vi "TangoEventsTest.vi"() -> ()   [LabVIEW 2009]
uses:
  tango_lv9/tango_vi.llb/tango.lvlib
  tango_lv9/tango_vi.llb/toShortScalar.vi
panel:
  in  "event timeout (ms)":i32=1000
  out "event timeout":bool=TRUE
  out "source":string
  out "quality":string
  out "Graphe déroulant 2":i16(graph)
  out "value":i16
  out "event error stack":string[](array[string])
  out "timestamp":string
  in  "unsubscribe 2":bool=TRUE
  in  "device name":string="tango/tangotest/1"
  in  "attribute name":string="short_scalar"
  # "EVENT SOURCE\n\nEVENT SUBSCRIPTION"
  # "EVENT HANDLER\n\nEVENT HANDLER"
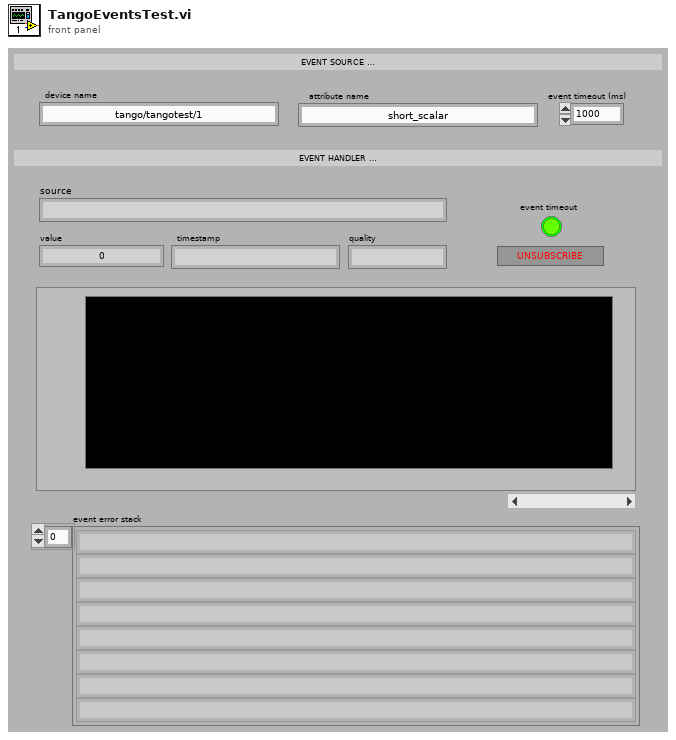
[diagram p1: front panel]
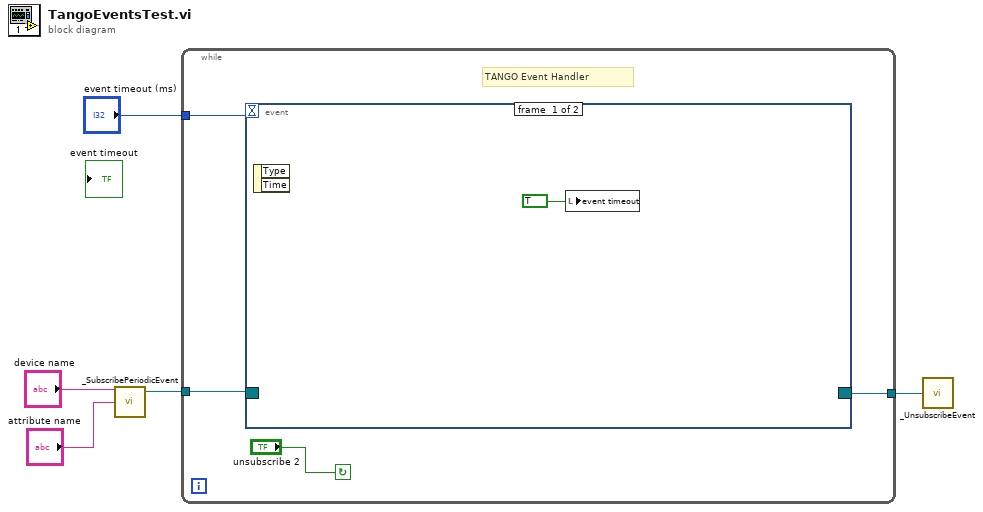
[diagram p0: block diagram]
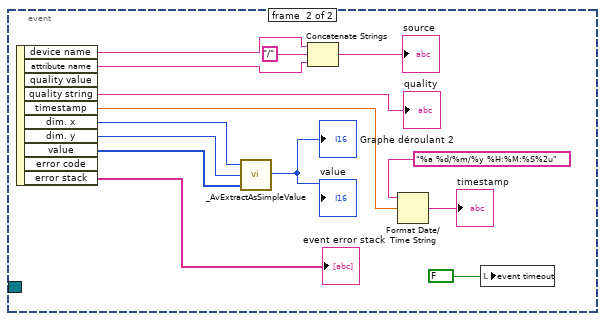
[diagram p2: hidden frame]
diagram:
  n1 = call "_SubscribePeriodicEvent.vi"("attribute name"="attribute name", "device name"="device name") -> ("refnum"=w3:refnum<event-registration>)  [unwired: 1 in, 2 out]
  n2 = while {
    tunnel: [w8] -> w4
    tunnel: "event timeout (ms)" -> [w7]
    tunnel: w3 -> [w6]
    stop <- "unsubscribe 2" continue-if-true
    # "TANGO Event Handler"
    n3 = event shown="[1] <attribute value>: User Event" {
      selector: w6 -> [_ _]
      dyn-events: [_ _] -> w8
      timeout: w7 -> [_ _]
      event #0 {
        n4 = event-data() -> ()  [unwired: 1 in, 2 out]
        n5 = local write "event timeout"(TRUE) -> ()
      }
      event #1 {
        n6 = event-data() -> ("device name"=w21:string, "attribute name"=w20:string, "quality string"=→"quality":string, "timestamp"=w11:dbl, "dim. x"=w17:i32, "dim. y"=w16:i32, "value"=w15:u8[], "error stack"=→"event error stack":string[])  [unwired: 1 in, 2 out]
        n7 = call-poly "_AvExtractAsSimpleValue.vi"("value_in"=w15, "dim_y"=w16, "dim_x"=w17) -> ("value_out"=→"Graphe déroulant 2" →"value":i16)  [unwired: 1 out]
        n8 = Concatenate Strings(w21, "/" ("chaîne"), w20) -> (→"source":string)
        n9 = Format Date/Time String(time format string (%c)="%a %d/%m/%y %H:%M:%S%2u" ("chaîne de format de l'heure (%c)"), seconds (now)=w11) -> (date/time string=→"timestamp":string)  [unwired: 1 in]
        n10 = local write "event timeout"(FALSE) -> ()
      }
    }
  }
  n11 = call "_UnsubscribeEvent.vi"("refnum"=w4) -> ()  [unwired: 2 out]
